vi "Power Meter Front Panel.vi"() -> ()   [LabVIEW 2009]
doc: "Front Panel for Newport 1830-C power meter."
uses:
  Global/GPIB Numbers.vi
  Newport 1830-C/Newport 1830-C.lvlib
panel:
  in  "AVG?":bool
  in  "Averaging Time":dbl[unit]=0.5
  in  "Read to Controls":bool
  out "Units":u16(ring) items=["W"=1, "dB"=2, "dBm"=3, "REL"=4]
  out "AVG":u16(ring) items=["Slow"=1, "Medium"=2, "Fast"=3]
  out "Run/Stop":u16(ring) items=["Stop", "Run"]
  out "ATTN":u16(ring) items=["Off", "On"]
  out "Local Lockout":u16(ring) items=["Off", "On"]
  out "Zero":u16(ring) items=["Off", "On"]
  out "Beeper":u16(ring) items=["Off", "On"]
  out "Backlight":u16(ring) items=["Off", "Low", "High"]
  out "Range":u16(ring) items=["Auto", "Lowest", "2", "3", "4", "5", "6", "7", "Highest"]
  out "Wavelength":dbl[unit]
  in  "Read Count":i32=1
  out "SI Power":string
  out "Power":dbl
  out "error code out":i32 format="%0.0f"
  in  "Read":bool caption="Read to Controls"
  in  "Read Power":bool
  in  "Set":bool
  in  "Run/Stop":u32(ring)=1 items=["Stop", "Run"]
  in  "Wavelength":dbl[unit]=8.200000000000001e-07
  in  "stop":bool
  in  "ATTN":u32(ring) items=["Off", "On"]
  in  "BKLT":u32(ring)=1 items=["Off", "Low", "High"]
  in  "Range":u32(ring) items=["Auto", "Lowest", "2", "3", "4", "5", "6", "7", "Highest"]
  in  "Beep":u32(ring) items=["Off", "On"]
  in  "AVG":u32(ring)=2 items=["Slow"=1, "Medium"=2, "Fast"=3]
  in  "Store\nReference":bool
  in  "Units":u32(ring)=1 items=["W"=1, "dB"=2, "mdB"=3, "REL"=4]
  in  "Zero":u32(ring) items=["Off", "On"]
  in  "Local":u32(ring) items=["Off", "On"]
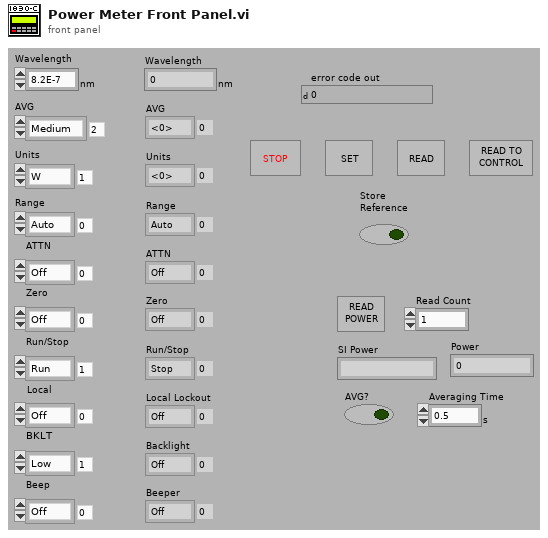
[diagram p1: front panel]
types:
  T1 = typedef "GPIB Type Def.ctl" = cluster{"Name":string, "bus":dbl, "GPIB":dbl, "GPIB as string":string, "byte":i32, "VISA Resource Name":refnum<visa-resource-name>}
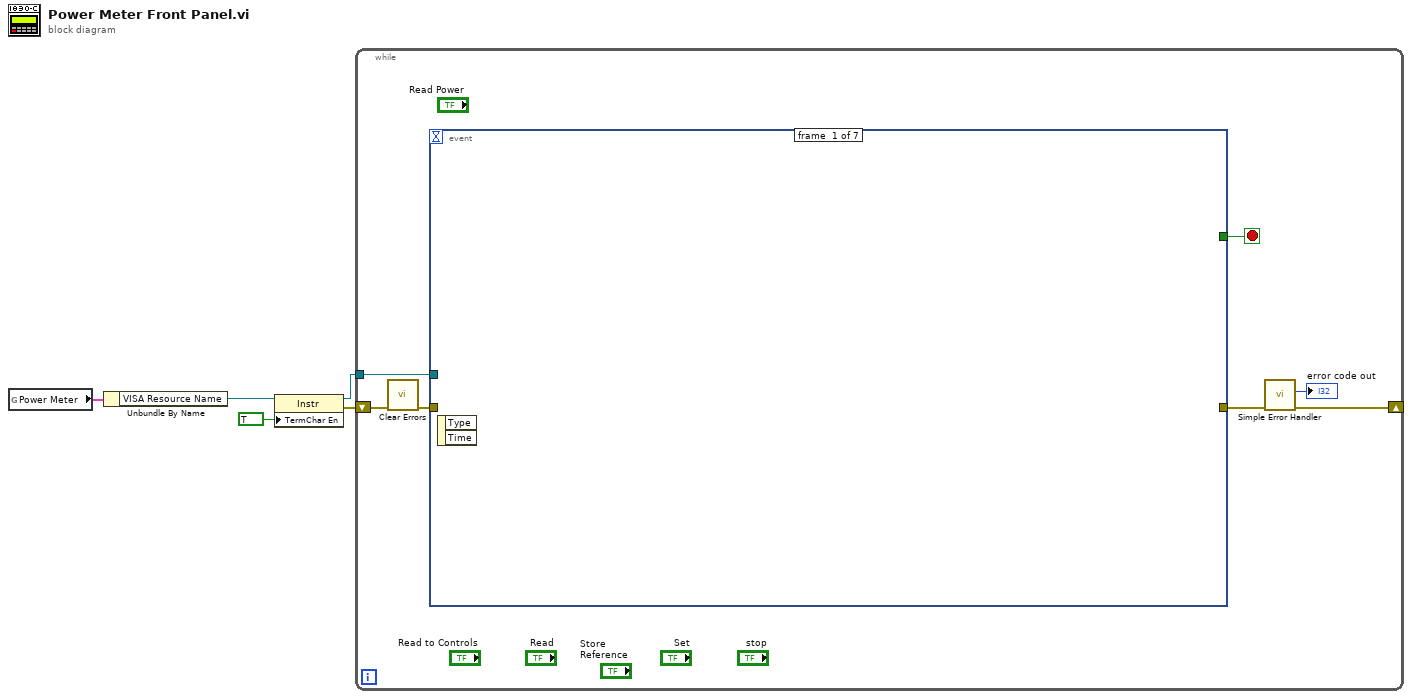
[diagram p0: block diagram]
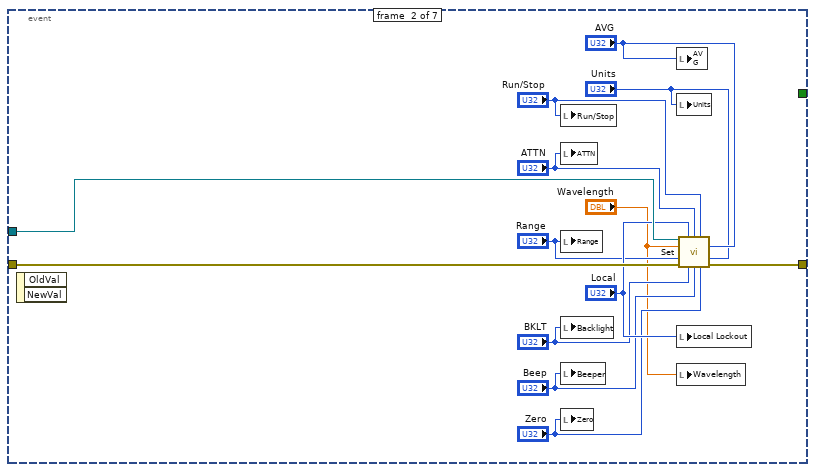
[diagram p2: hidden frame]
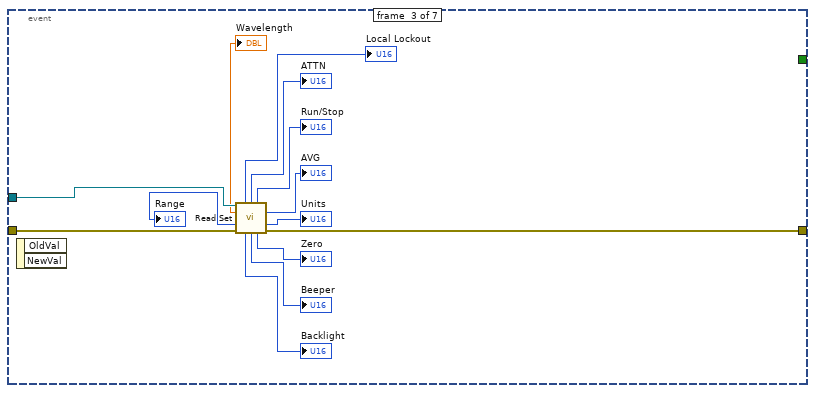
[diagram p3: hidden frame]
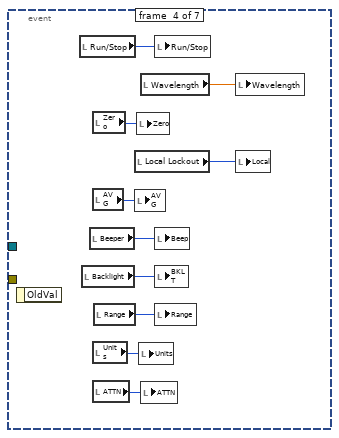
[diagram p4: hidden frame]
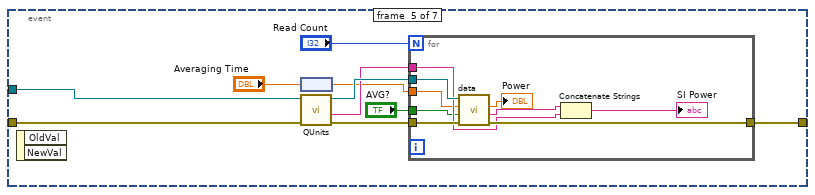
[diagram p5: hidden frame]
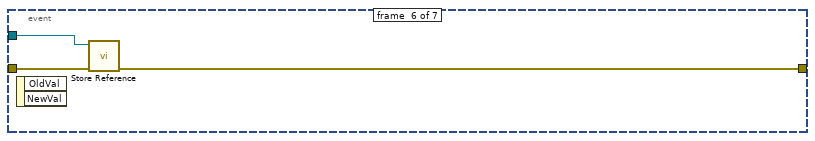
[diagram p6: hidden frame]
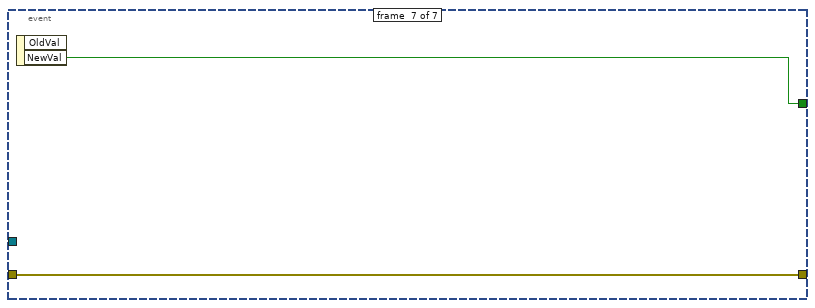
[diagram p7: hidden frame]
diagram:
  n1 = global read "GPIB Numbers.vi" "Power Meter"() -> (w2:T1)
  n2 = Unbundle By Name(w2) -> ("VISA Resource Name"=w1:refnum<visa-resource-name>)
  n3 = property class="Instr"(reference=w1, "TermChar En"=TRUE ("Message Based Settings:Termination Character Enable")) -> (reference out=w5:refnum<visa-resource-name>, error out=w4:errorcluster)  [unwired: 1 in]
  n4 = while {
    shift-right: [w12] -> _
    shift-left: w4 -> [w11]
    tunnel: w5 -> [w7]
    stop <- w9 stop-if-true
    n5 = call <vilib>:"Clear Errors.vi"("error in (no error)"=w11) -> ("error out"=w6:errorcluster)  [unwired: 6 in]
    n6 = event shown="[4] \"Read Power\": Value Change" {
      selector: _ -> [_ _ _ _ _ _ _]
      dyn-events: _ -> [_ _ _ _ _ _ _]
      timeout: _ -> [_ _ _ _ _ _ _]
      tunnel: w7 -> [_ w24 w38 _ w57 w70 _]
      tunnel: w6 -> [_ w25 w37 _ w56 w69 w71]
      tunnel: [_ w23 w36 _ w58 w68 w71] -> w10
      tunnel: [_ _ _ _ _ _ w72] -> w9
      event #0 {
        n7 = event-data() -> ()  [unwired: 1 in, 2 out]
      }
      event #1 {
        n8 = event-data() -> ()  [unwired: 1 in, 2 out]
        n9 = local write "Run/Stop"("Run/Stop") -> ()
        n10 = local write "ATTN"("ATTN") -> ()
        n11 = local write "Range"("Range") -> ()
        n12 = local write "Backlight"("BKLT") -> ()
        n13 = local write "Beeper"("Beep") -> ()
        n14 = local write "Zero"("Zero") -> ()
        n15 = local write "AVG"("AVG") -> ()
        n16 = local write "Units"("Units") -> ()
        n17 = local write "Local Lockout"("Local") -> ()
        n18 = local write "Wavelength"("Wavelength") -> ()
        n19 = call "Set.vi"("VISA resource name"=w24, "Local Lockout (0:1)"="Local", "ATTN (0:1)"="ATTN", "Run/Stop (1:0)"="Run/Stop", "Wavelength (nnnn)"="Wavelength", "AVG (1:3)"="AVG", "Range (0-Auto,1:8)"="Range", "Units (1:4)"="Units", "error in (no error)"=w25, "Backlight (0:2)"="BKLT", "Beeper (0:1)"="Beep", "Zero (0:1)"="Zero") -> ("error out"=w23:errorcluster)  [unwired: 2 in, 1 out]
      }
      event #2 {
        n20 = event-data() -> ()  [unwired: 1 in, 2 out]
        n21 = call "Read Set.vi"("VISA resource name"=w38, "error in (no error)"=w37) -> ("Local Lockout"=→"Local Lockout":u32, "ATTN"=→"ATTN":u32, "Run/Stop"=→"Run/Stop":u32, "Wavelength (nnnn)"=→"Wavelength":dbl[unit], "AVG"=→"AVG":u32, "Range (1:8)"=→"Range":u32, "Units"=→"Units":u32, "Backlight"=→"Backlight":u32, "Beeper"=→"Beeper":u32, "Zero"=→"Zero":u32, "error out"=w36:errorcluster)  [unwired: 2 in, 1 out]
      }
      event #3 {
        n22 = event-data() -> ()  [unwired: 1 in, 1 out]
        n23 = local read "Run/Stop"() -> (w47:u16)
        n24 = local read "Backlight"() -> (w41:u16)
        n25 = local read "Beeper"() -> (w40:u16)
        n26 = local read "Zero"() -> (w39:u16)
        n27 = local read "AVG"() -> (w45:u16)
        n28 = local read "Units"() -> (w43:u16)
        n29 = local read "ATTN"() -> (w46:u16)
        n30 = local read "Range"() -> (w42:u16)
        n31 = local read "Local Lockout"() -> (w48:u16)
        n32 = local write "AVG"(w45) -> ()
        n33 = local write "Zero"(w39) -> ()
        n34 = local write "Units"(w43) -> ()
        n35 = local read "Wavelength"() -> (w44:dbl[unit])
        n36 = local write "ATTN"(w46) -> ()
        n37 = local write "Run/Stop"(w47) -> ()
        n38 = local write "Beep"(w40) -> ()
        n39 = local write "BKLT"(w41) -> ()
        n40 = local write "Range"(w42) -> ()
        n41 = local write "Wavelength"(w44) -> ()
        n42 = local write "Local"(w48) -> ()
      }
      event #4 {
        n43 = event-data() -> ()  [unwired: 1 in, 2 out]
        n44 = node("Averaging Time") -> (w49:dbl)
        n45 = call "QUnits.vi"("error in (no error)"=w56, "VISA resource name"=w57) -> ("error out"=w54:errorcluster, "Unit Label"=w52:string, "VISA resource name out"=w55:refnum<visa-resource-name>)  [unwired: 6 in, 1 out]
        n46 = for {
          N: "Read Count" -> [_]
          tunnel: w55 -> [w67]
          tunnel: w54 -> [w66]
          tunnel: [w65] -> w58
          tunnel: w52 -> [w63]
          tunnel: w49 -> [w60]
          tunnel: "AVG?" -> [w59]
          n47 = call "data.vi"("error in (no error)"=w66, "AVG?"=w59, "Averaging Time"=w60, "VISA resource name"=w67) -> ("error out"=w65:errorcluster, "SI"=w62:string, "output"=→"Power":dbl)  [unwired: 4 in, 1 out]
          n48 = Concatenate Strings(w62, w63) -> (→"SI Power":string)
        }
      }
      event #5 {
        n49 = event-data() -> ()  [unwired: 1 in, 2 out]
        n50 = call "Store Reference.vi"("error in (no error)"=w69, "VISA resource name"=w70) -> ("error out"=w68:errorcluster)  [unwired: 8 in, 1 out]
      }
      event #6 {
        n51 = event-data() -> ("NewVal"=w72:bool)  [unwired: 1 in, 1 out]
      }
    }
    n52 = call <vilib>:"Simple Error Handler.vi"("error in (no error)"=w10) -> ("code out"=→"error code out":i32, "error out"=w12:errorcluster)  [unwired: 4 in, 3 out]
  }
